vi "test Segmented Upload Visible String.vi"(11 "Test Case In":refnum<class "Tests SDO Manager.lvclass">) -> (0 "error out":errorcluster, 3 "Test Case Out":refnum<class "Tests SDO Manager.lvclass">)   [LabVIEW 2020, in "Tests SDO Manager.lvclass"]
uses:
  Tests SDO Manager.lvclass
  Tests SDO Manager.lvclass/Tests SDO Manager.ctl
  Simulated CANopen Node/Simulated CANopen Node.lvclass
  D:/git/HAL/Source/Interfaces/IInstrument/IInstrument.lvclass
  D:/git/HAL/Source/Interfaces/IClose/IClose.lvclass
  D:/git/HAL/Source/Interfaces/IInitialize/IInitialize.lvclass
  D:/git/CANopen-LabVIEW/tests/Simulated CANopen Node/Simulated CANopen Node.lvclass
  D:/git/HAL/Source/Interfaces/ICommunicate/ICommunicate.lvclass
  source/Logging/Logger/Logger.lvclass
  C:/Program Files/National Instruments/LabVIEW 2026/vi.lib/ActorFramework/Actor/Actor.lvclass
  D:/git/CANopen-LabVIEW/source/Logging/Logger/Logger.lvclass
  4993e8ee-a06a-463a-9684-69129f64d5ce.vi
  source/SDO Manager/SDO Manager/SDO Manager/SDO Manager.lvclass
  source/Logging/Log Level.vi
  source/Logging/CANopen Logging.lvlib
  <vilib>/ActorFramework/Actor/Actor.lvclass
  <vilib>/ActorFramework/Stop Msg/Stop Msg.lvclass
  source/SDO Manager/SDO Manager/SDO Manager/Upload Visible String.vi
  source/SDO Manager/SDO Manager/SDO Transfer/SDO abort code.ctl
  source/SDO Manager/SDO Manager/SDO Transfer/SDO Transfer.lvclass
  source/Typedefs/SDO Result.ctl
panel:
  out "SDO Result":T1={"Success"=FALSE, "SDO abort code"={"Null"=TRUE, "Value"=84082688}, "Data"={"Null"=TRUE, "Data"=[]}} {"SDO abort code"."Value" items=["Toggle bit not allowed"=84082688, "SDO protocol timed out"=84148224, "Client/server command specifier not valid or unknown"=84148225, "Invalid block size (block mode only)"=84148226, "Invalid sequence number (block mode only)"=84148227, "CRC error (block mode only)"=84148228, "Out of memory"=84148229, "Attempt to read a write only object"=100728833, "Attempt to write a read only object"=100728834, "Object does not exist in the object dictionary"=100794368, "Object cannot be mapped to the PDO"=100925505, "The number and length of the objects to be mapped would exceed PDO length"=100925506, "General parameter incompatibility reason"=100925507, "General internal incompatibility in the device"=100925511, "Access failed due to an hardware error"=101056512, "Data type does not match, length of service parameter does not match"=101122064, "Data type does not match, length of service parameter too high"=101122066, "Data type does not match, length of service parameter too low"=101122067, "Sub-index does not exist"=101253137, "Invalid value for parameter (download only)"=101253168, "Value of parameter written too high (download only)"=101253169, "Value of parameter written too low (download only)"=101253170, "Maximum value is less than minimum value"=101253174, "Resource not available: SDO connection"=101318691, "General error"=134217728, "Data cannot be transferred or stored to the application"=134217760, "Data cannot be transferred or stored to the application because of local control"=134217761, "Data cannot be transferred or stored to the application because of the present device stable"=134217762, "Object dictionary dynamic generation fails or no object dictionary is present (e.g. object dictionary is generated from file and generation fails because of an file error)"=134217763, "No data available"=134217764]; "Data"."Data" format="%02x"}
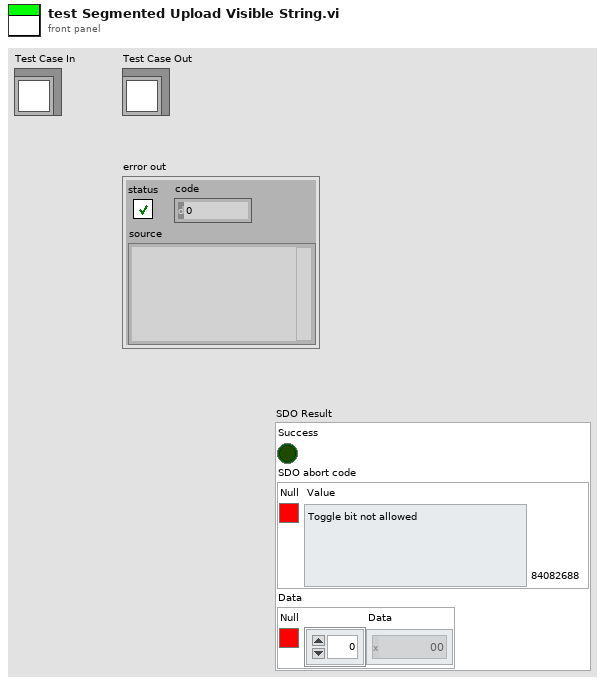
[diagram p1: front panel]
types:
  T1 = typedef "CANopen.lvlib/SDO Manager.lvlib/SDO Transfer.lvclass/SDO Result.ctl" = cluster{"Success":bool, "SDO abort code":cluster{"Null":bool, "Value":T2}, "Data":cluster{"Null":bool, "Data":u8[]}}
  T2 = typedef "CANopen.lvlib/SDO Manager.lvlib/SDO Transfer.lvclass/SDO abort code.ctl" = u32
  T3 = cluster{"Node-ID":u8, "Multiplexer":cluster{"Index":u16, "Sub-Index":u8}}
  T4 = enum16{"Error", "Warn", "Info", "Debug", "Trace"}
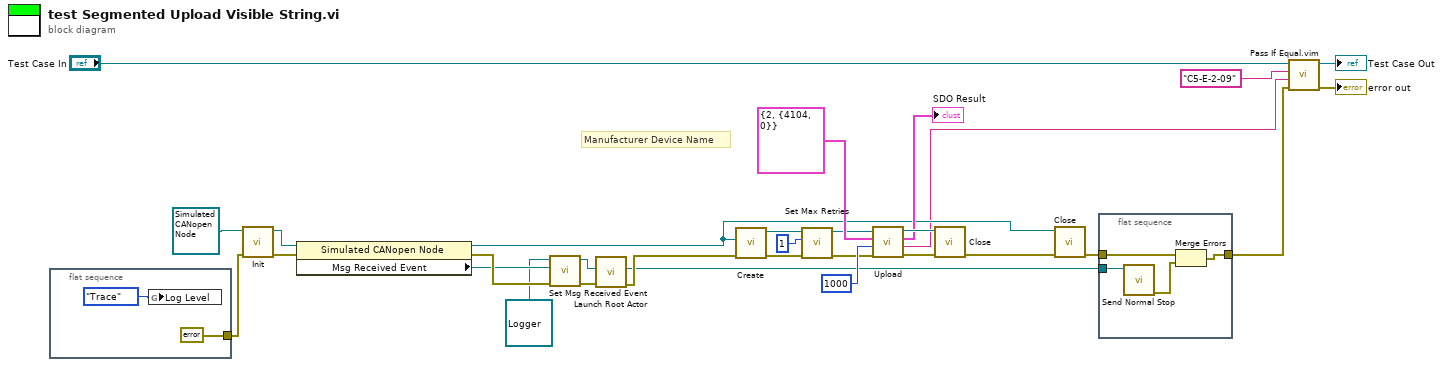
[diagram p0: block diagram]
diagram:
  # "Manufacturer Device Name"
  n1 = flat-sequence {
    tunnel: [errorcluster {"status"=FALSE, "code"=0, "source"=""} ("error constant")] -> w3
    frame #0 {
      n2 = global write "Log Level.vi" "Log Level"(T4."Trace" ("Log Level")) -> ()
    }
  }
  n3 = call-dynamic "Init.vi"("error in"=w3, "Simulated CANopen Node in"=refnum<class "Simulated CANopen Node.lvclass"> refnum ("Simulated CANopen Node.lvclass")) -> ("error out"=w19:errorcluster, "Simulated CANopen Node out"=w18:refnum<class "Simulated CANopen Node.lvclass">)  [unwired: 8 in]
  n4 = property class="Simulated CANopen Node"(reference=w18, error in=w19) -> (reference out=w2:refnum<class "Simulated CANopen Node.lvclass">, error out=w17:errorcluster, "Msg Received Event"=w16:refnum<user-event>)
  n5 = call "Set Msg Received Event.vi"("error in"=w17, "Msg Received Event"=w16, "Logger in"=refnum<class "Logger.lvclass"> refnum) -> ("error out"=w21:errorcluster, "Logger out"=w20:refnum<class "Logger.lvclass">)  [unwired: 7 in]
  n6 = call <vilib>:"Launch Root Actor.vi"("error in (no error)"=w21, "Actor"=w20) -> ("error out"=w15:errorcluster, "Actor's Enqueuer"=w12:refnum<class "Message Enqueuer.lvclass">)  [unwired: 8 in]
  n7 = call "Create.vi"("Error In"=w15, "ICommunicate"=w2) -> ("Error Out"=w10:errorcluster, "SDO Manager"=w9:refnum<class "SDO Manager.lvclass">)  [unwired: 8 in]
  n8 = call "Set Max Retries.vi"("error in"=w10, "Max Retries"=u8 1, "SDO Manager in"=w9) -> ("error out"=w7:errorcluster, "SDO Manager out"=w8:refnum<class "SDO Manager.lvclass">)  [unwired: 7 in]
  n9 = call-poly "Upload.vi"("Error In"=w7, "Retry Delay (ms)"=1000 ("Timeout"), "Parameters"=T3 {"Node-ID"=2, "Multiplexer"={"Index"=4104, "Sub-Index"=0}}, "SDO Manager in"=w8) -> ("Error Out"=w25:errorcluster, "Visible String"=w1:string, "SDO Result"=→"SDO Result":T1, "SDO Manager out"=w24:refnum<class "SDO Manager.lvclass">)  [unwired: 4 in]
  n10 = call "Close.vi"("Error In"=w25, "SDO Manager"=w24) -> ("Error Out"=w27:errorcluster)  [unwired: 8 in, 1 out]
  n11 = call-dynamic "Close.vi"("error in"=w27, "Simulated CANopen Node in"=w2) -> ("error out"=w13:errorcluster)  [unwired: 8 in, 1 out]
  n12 = flat-sequence {
    tunnel: w13 -> [w33]
    tunnel: w12 -> [w36]
    tunnel: [w34] -> w11
    frame #0 {
      n13 = call <vilib>:"Send Normal Stop.vi"("Message Enqueuer"=w36) -> ("error out"=w35:errorcluster)  [unwired: 10 in]
      n14 = Merge Errors(w33, w35) -> (w34:errorcluster)
    }
  }
  n15 = call "Pass If Equal.vim"("error in (no error)"=w11, "Actual"=w1, "Expected"="C5-E-2-09", "LUnit Test Case In"="Test Case In") -> ("error out"=→"error out":errorcluster, "LUnit Test Case Out"=→"Test Case Out":refnum<class "Tests SDO Manager.lvclass">)  [unwired: 6 in]
